vi "Load Config.vi"(8 "error in (no error)":errorcluster, 10 "JSON":string, 11 "HistorianCharting in":refnum<class "HistorianCharting.lvclass">) -> (0 "error out":errorcluster, 3 "HistorianCharting out":refnum<class "HistorianCharting.lvclass">)   [LabVIEW 2020, in "VolatusGUIElements.lvlib" / "HistorianCharting.lvclass"]
uses:
  HistorianCharting.lvclass
  JSON.ctl
  HistorianCharting.lvclass/HistorianCharting.ctl
  e13d5b10-92df-4313-bdba-81b966c83aec.vi
  <vilib>/JDP Science/JSONtext/JSON text to Variant.vi
  <vilib>/JDP Science/JSONtext/LVClass Serializer/JSONtext LVClass Serializer.lvclass
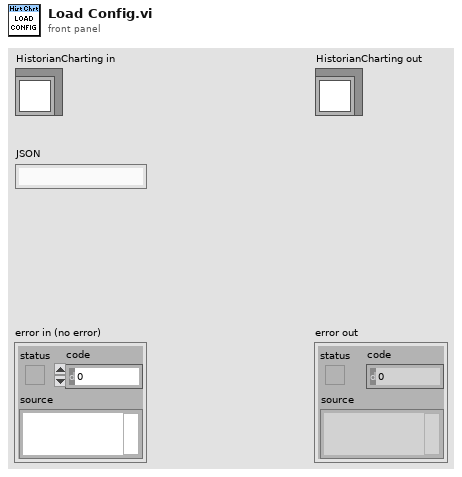
[diagram p1: front panel]
types:
  T1 = typedef "VolatusGUIElements.lvlib/HistorianCharting.lvclass/JSON.ctl" = cluster{"Managed":bool, "Redraw Period":dbl}
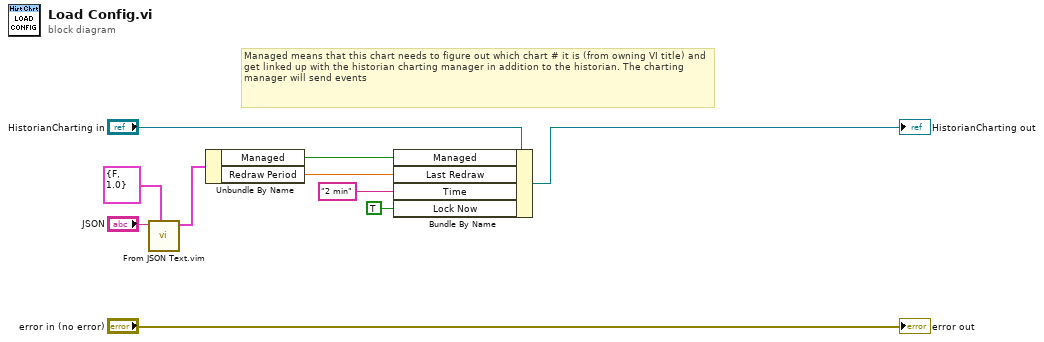
[diagram p0: block diagram]
diagram:
  # "Managed means that this chart needs to figure out which chart # it is (from owning VI title) and get linked up with the historian charting manager in addition to the historian. The charting manager will send events"
  n1 = call "From JSON Text.vim"("Data Type and Default Value"=T1 {"Managed"=FALSE, "Redraw Period"=1.0} ("JSON"), "JSON"="JSON") -> ("Data out"=w5:T1)  [unwired: 8 in, 1 out]
  n2 = Unbundle By Name(w5) -> ("Managed"=w4:bool, "Redraw Period"=w3:dbl)
  n3 = Bundle By Name(cluster="HistorianCharting in", "Managed"=w4, "Last Redraw"=w3, "Time"="2 min" ("Plot Config.Time"), "Lock Now"=TRUE ("Plot Config.Lock Now")) -> (→"HistorianCharting out":refnum<class "HistorianCharting.lvclass">)
  "error out" <- "error in (no error)"
